vi "获取Y轴信息.vi"(9 "错误输入（无错误）":errorcluster, 10 "VISA资源名称":refnum<visa-resource-name>) -> (1 "错误输出":errorcluster, 2 "VISA资源名称输出":refnum<visa-resource-name>, 4 "YZEro":dbl, 5 "YMUlt":dbl, 6 "YUNit":string, 7 "YOFf":dbl)   [LabVIEW 2017]
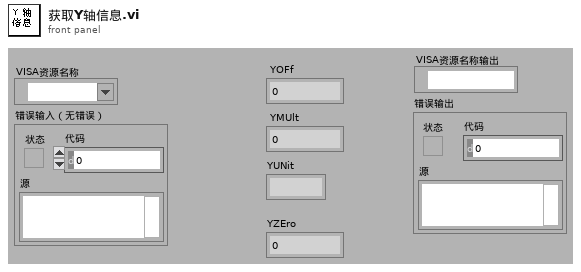
[diagram p1: front panel]
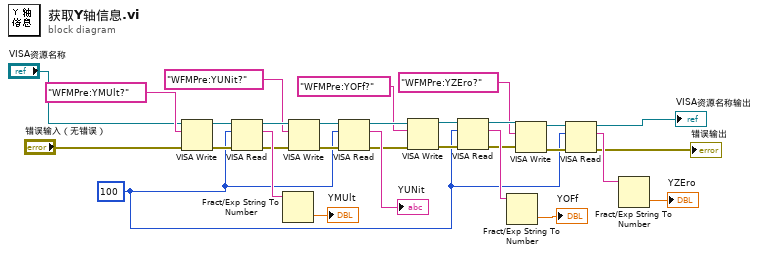
[diagram p0: block diagram]
diagram:
  w3 = u32 100 ("字节总数")
  n1 = VISA Write(VISA resource name="VISA资源名称", write buffer="WFMPre:YMUlt?" ("写入缓冲区"), error in (no error)="错误输入（无错误）") -> (VISA resource name out=w30:refnum<visa-resource-name>, error out=w29:errorcluster)  [unwired: 1 out]
  n2 = VISA Read(VISA resource name=w30, byte count=w3, error in (no error)=w29) -> (VISA resource name out=w24:refnum<visa-resource-name>, read buffer=w27:string, error out=w23:errorcluster)  [unwired: 1 out]
  n3 = Fract/Exp String To Number(string=w27) -> (number=→"YMUlt":dbl)  [unwired: 3 in, 1 out]
  n4 = VISA Write(VISA resource name=w24, write buffer="WFMPre:YUNit?" ("写入缓冲区"), error in (no error)=w23) -> (VISA resource name out=w26:refnum<visa-resource-name>, error out=w25:errorcluster)  [unwired: 1 out]
  n5 = VISA Read(VISA resource name=w26, byte count=w3, error in (no error)=w25) -> (VISA resource name out=w18:refnum<visa-resource-name>, read buffer=→"YUNit":string, error out=w17:errorcluster)  [unwired: 1 out]
  n6 = VISA Write(VISA resource name=w18, write buffer="WFMPre:YOFf?" ("写入缓冲区"), error in (no error)=w17) -> (VISA resource name out=w20:refnum<visa-resource-name>, error out=w19:errorcluster)  [unwired: 1 out]
  n7 = VISA Read(VISA resource name=w20, byte count=w3, error in (no error)=w19) -> (VISA resource name out=w11:refnum<visa-resource-name>, read buffer=w15:string, error out=w10:errorcluster)  [unwired: 1 out]
  n8 = Fract/Exp String To Number(string=w15) -> (number=→"YOFf":dbl)  [unwired: 3 in, 1 out]
  n9 = VISA Write(VISA resource name=w11, write buffer="WFMPre:YZEro?" ("写入缓冲区"), error in (no error)=w10) -> (VISA resource name out=w14:refnum<visa-resource-name>, error out=w13:errorcluster)  [unwired: 1 out]
  n10 = VISA Read(VISA resource name=w14, byte count=w3, error in (no error)=w13) -> (VISA resource name out=→"VISA资源名称输出":refnum<visa-resource-name>, read buffer=w12:string, error out=→"错误输出":errorcluster)  [unwired: 1 out]
  n11 = Fract/Exp String To Number(string=w12) -> (number=→"YZEro":dbl)  [unwired: 3 in, 1 out]
